vi "WPI_RelayDoesDevRefExist.vi"(0 "RelayDevRefArray":T1[](array[typedef]), 7 "RelayDevRef":T1={"DevStatus"={"status"=FALSE, "code"=0, "source"=""}, "Relay Channel"=enum."Relay 2", "Relay Direction"=enum."Both directions"}) -> (4 "index":i32, 8 "exists":bool)   [LabVIEW 2017]
doc: "This is used to find the index of a DevRef within an array of DevRefs."
uses:
  <vilib>/Rock Robotics/WPI/Relay/WPI_RelayDevRef.ctl
  <vilib>/Rock Robotics/SystemInterfaces/DIO/FPGA_DIORelayChannel.ctl
  <vilib>/Rock Robotics/WPI/Relay/WPI_RelayDirection.ctl
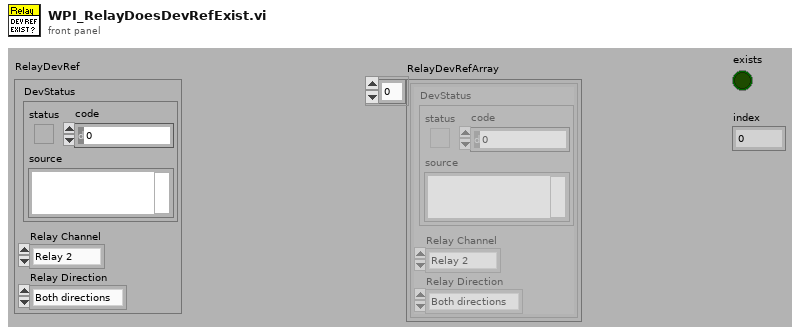
[diagram p1: front panel]
types:
  T1 = typedef "WPI_RelayDevRef.ctl" = cluster{"DevStatus":errorcluster, "Relay Channel":T2, "Relay Direction":T3}
  T2 = typedef "FPGA_DIORelayChannel.ctl" = enum8{"Relay 0", "Relay 1", "Relay 2", "Relay 3", "Invalid"}
  T3 = typedef "WPI_RelayDirection.ctl" = enum16{"Both directions", "Forward only", "Reverse only"}
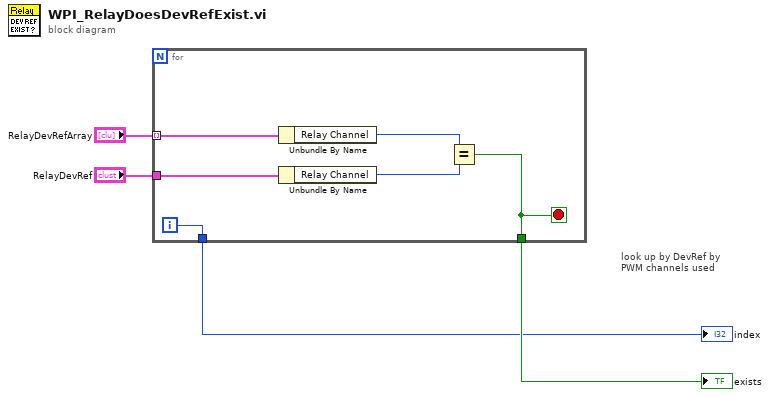
[diagram p0: block diagram]
diagram:
  # "look up by DevRef by PWM channels used"
  n1 = for {
    tunnel: "RelayDevRefArray" -> [w10] mode=indexing
    tunnel: "RelayDevRef" -> [w9]
    tunnel: [w8] -> w2
    tunnel: [w7] -> w1
    i -> [w7]
    stop <- w8 stop-if-true
    n2 = Unbundle By Name(w10) -> ("Relay Channel"=w6:T2)
    n3 = Unbundle By Name(w9) -> ("Relay Channel"=w5:T2)
    n4 = Equal?(x=w6, y=w5) -> (x = y?=w8:bool)
  }
  "exists" <- w2
  "index" <- w1
